vi "PH_PowerUnit_BaseClass.calc Status.vi"(0 "VI in":refnum<vi>, 5 "error in (no error)":errorcluster) -> (14 "VI out":refnum<vi>, 16 "PU Status":T1 items=["no info", "off/false/out", "on/true/in", "Failure", "Alarm", "Status 1", "Status 2", "Status 3"], 19 "error out":errorcluster)   [LabVIEW 2014, in "PH_PowerUnit_BaseClass.lvlib"]
uses:
  PH_PowerUnit_BaseClass.lvlib
  PH_StatusHandler/PH_StatusHandler.Status.ctl
  PH_StatusHandler/PH_StatusHandler.lvlib
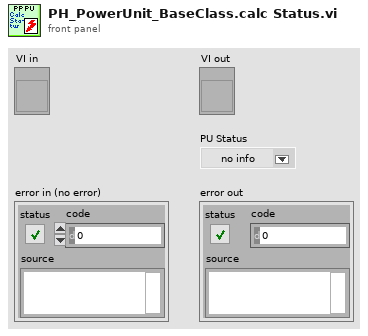
[diagram p1: front panel]
types:
  T1 = typedef "PH_StatusHandler.lvlib/PH_StatusHandler.Status.ctl" = i16
  T2 = typedef "PH_PowerUnit_BaseClass.lvlib/PH_PowerUnit_BaseClass.i attribute.ctl" = cluster{"Constructor finished":bool, "PU":cluster{"In use":bool, "Service ID in use":i32, "GUI Ref":refnum<vi>}, "Enabling":cluster{"State":T3, "GUI Ref":refnum<vi>}, "Timing":cluster{"Last Shot":dbl, "Time between Shots [Sec]":dbl, "Waiting Time over?":bool, "Service ID Waiting Time":i32, "GUI Ref":refnum<vi>, "Instance":cluster{"Status":T1, "linked?":bool, "GUI Ref":refnum<vi>}}, "Sequencer":cluster{"SM State":string, "GUI Ref":refnum<vi>, "linked":bool}, "Subscribed Trendmssgs":cluster{"Tagname":string, "Status":T1, "linked?":bool, "Shot Condition":T1, "GUI Ref":refnum<vi>}[], "PP PU":T4, "Default Voltage (V)":dbl, "GUI Refs":T5, "PSDB data":cluster{"Shot Voltage [V]":dbl, "State TO SM":T6, "Write 2 early":bool}, "State TO SM":T6}
  T3 = typedef "PH_SystemInformation.lvlib/PH_SystemInformationEnabling State.ctl" = i32
  T4 = typedef "PH_PP_Common.lvlib/PH_PP_Common.PUs.ctl" = enum16{"no Info", "PA-19mm-1", "PA-19mm-2", "PA-45mm-PILC", "PA-45mm-MAIN", "MA-PU-1", "MA-PU-2", "MA-PU-3", "MA-PU-4", "MA-PU-5", "MA-PU-6", "MA-FR", "MA-PILC", "PA-45mm-DP"}
  T5 = typedef "PH_PowerUnit_BaseClass.lvlib/PH_PowerUnit_BaseClass.GUI Refs.ctl" = cluster{"Delete Inst":refnum<vi>, "State TO SM":refnum<vi>, "State SM":refnum<vi>, "Fire":refnum<vi>}
  T6 = typedef "PH_PowerUnit_BaseClass.lvlib/PH_PowerUnit_BaseClass.SM States.ctl" = enum16{".", "Stand by", "Switch PU on", "Configure", "Set Default Voltage", "Set STANDBY", "Set READY", "Wait for Shot Cmd", "Open Dump Rods", "Open Ross Relais", "Close Ross Relais", "Switch PSU on", "Switch PSU off", "Charge", "Switch GD Channel on", "Close Dump Rods", "Rods-TO", "RR-TO", "PSU-TO", "Trigger-TO"}
  T7 = cluster{"Tagname":string, "Status":T1, "linked?":bool, "Shot Condition":T1, "GUI Ref":refnum<vi>}[]
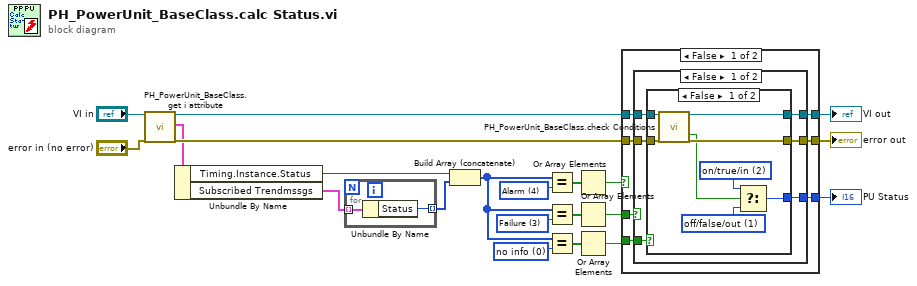
[diagram p0: block diagram]
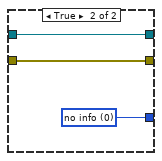
[diagram p2: hidden frame]
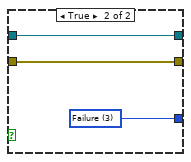
[diagram p3: hidden frame]
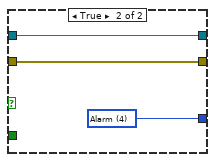
[diagram p4: hidden frame]
diagram:
  w21 = T1 4 items=["no info", "off/false/out", "on/true/in", "Failure", "Alarm", "Status 1", "Status 2", "Status 3"] ("Status")
  w20 = T1 3 items=["no info", "off/false/out", "on/true/in", "Failure", "Alarm", "Status 1", "Status 2", "Status 3"] ("Status")
  w19 = T1 0 items=["no info", "off/false/out", "on/true/in", "Failure", "Alarm", "Status 1", "Status 2", "Status 3"] ("Status")
  n1 = call "PH_PowerUnit_BaseClass.get i attribute.vi"("i ref in"="VI in", "error in (no error)"="error in (no error)") -> ("i ref out"=w17:refnum<vi>, "i attribute"=w7:T2, "error out"=w15:errorcluster)  [unwired: 15 in]
  n2 = Unbundle By Name(w7) -> ("Timing.Instance.Status"=w2:T1, "Subscribed Trendmssgs"=w1:T7)
  n3 = for {
    tunnel: w1 -> [w23] mode=indexing
    tunnel: [w22] -> w3 mode=indexing
    n4 = Unbundle By Name(w23) -> ("Status"=w22:T1)
  }
  n5 = Build Array (concatenate)(w2, w3) -> (w4:T1[])
  n6 = Equal?(x=w4, y=w21) -> (x = y?=w8:bool[])
  n7 = Equal?(x=w4, y=w20) -> (x = y?=w14:bool[])
  n8 = Equal?(x=w4, y=w19) -> (x = y?=w9:bool[])
  n9 = Or Array Elements(Boolean array=w8) -> (logical OR=w10:bool)
  n10 = Or Array Elements(Boolean array=w14) -> (logical OR=w11:bool)
  n11 = Or Array Elements(Boolean array=w9) -> (logical OR=w12:bool)
  n12 = case shown="False" w10 {
    tunnel: [w30 w53] -> w13
    tunnel: w11 -> [w29 _]
    tunnel: w12 -> [w28 _]
    tunnel: w15 -> [w27 w51]
    tunnel: [w26 w51] -> w16
    tunnel: w17 -> [w25 w52]
    tunnel: [w24 w52] -> w18
    frame False {
      n13 = case shown="False" w29 {
        tunnel: [w36 w50] -> w30
        tunnel: w28 -> [w35 _]
        tunnel: w27 -> [w34 w48]
        tunnel: [w33 w48] -> w26
        tunnel: w25 -> [w32 w49]
        tunnel: [w31 w49] -> w24
        frame False {
          n14 = case shown="False" w35 {
            tunnel: [w40 w47] -> w36
            tunnel: w34 -> [w44 w45]
            tunnel: [w43 w45] -> w33
            tunnel: w32 -> [w42 w46]
            tunnel: [w41 w46] -> w31
            frame False {
              w38 = T1 1 items=["no info", "off/false/out", "on/true/in", "Failure", "Alarm", "Status 1", "Status 2", "Status 3"] ("f")
              w39 = T1 2 items=["no info", "off/false/out", "on/true/in", "Failure", "Alarm", "Status 1", "Status 2", "Status 3"] ("Device Status")
              n15 = call "PH_PowerUnit_BaseClass.check Conditions.vi"("VI in"=w42, "error in (no error)"=w44) -> ("VI out"=w41:refnum<vi>, "Ready to switch PU on"=w37:bool, "error out"=w43:errorcluster)  [unwired: 14 in, 1 out]
              n16 = Select(t=w39, s=w37, f=w38) -> (s? t:f=w40:T1)
            }
            frame True {
              w47 = T1 0 items=["no info", "off/false/out", "on/true/in", "Failure", "Alarm", "Status 1", "Status 2", "Status 3"] ("Device Status")
            }
          }
        }
        frame True {
          w50 = T1 3 items=["no info", "off/false/out", "on/true/in", "Failure", "Alarm", "Status 1", "Status 2", "Status 3"] ("Device Status")
        }
      }
    }
    frame True {
      w53 = T1 4 items=["no info", "off/false/out", "on/true/in", "Failure", "Alarm", "Status 1", "Status 2", "Status 3"] ("Device Status")
    }
  }
  "VI out" <- w18
  "error out" <- w16
  "PU Status" <- w13
